vi "Close DSF Config Data.vi"(6 "version (no change)":T1, 8 "error in (no error)":errorcluster, 10 "write file if changed (T)":bool=TRUE, 11 "refnum":T2) -> (0 "error out":errorcluster, 3 "file path":path)   [LabVIEW 2017, in "DSF Configuration API.lvlib"]
doc: "Writes data to the platform-independent configuration file identified by <B>refnum</B> and then closes the reference to that file."
uses:
  DSF Configuration API.lvlib
  Controls/DSF Config Data RefNum.ctl
  Controls/Version Info.ctl
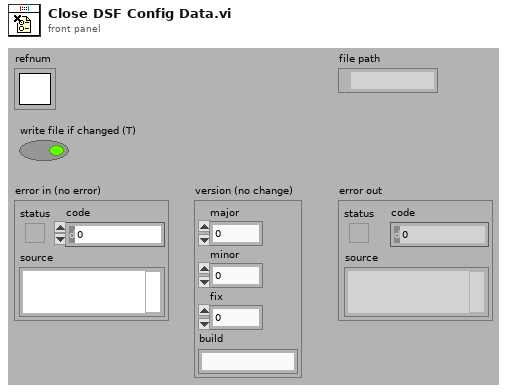
[diagram p1: front panel]
types:
  T1 = typedef "DSF Configuration API.lvlib/Version Info.ctl" = cluster{"major":u32, "minor":u32, "fix":u32, "build":string}
  T2 = typedef "DSF Configuration API.lvlib/DSF Config Data RefNum.ctl" = refnum<k1>
  T3 = typedef "DSF Configuration API.lvlib/Config Queue.ctl" = refnum<queue>
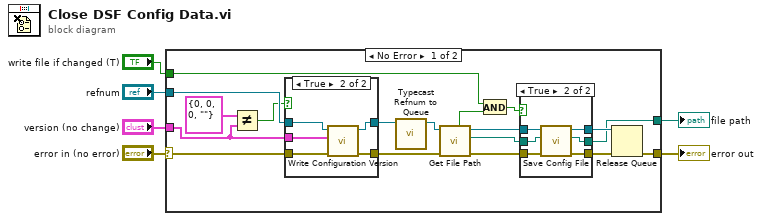
[diagram p0: block diagram]
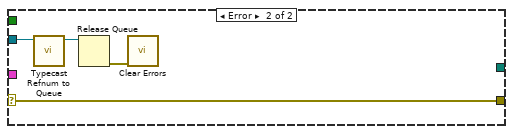
[diagram p4: hidden frame]
diagram:
  n1 = case shown="No Error" "error in (no error)" {
    selector: "error in (no error)" -> [w21 w44]
    tunnel: "refnum" -> [w11 w43]
    tunnel: "write file if changed (T)" -> [w23 _]
    tunnel: [w18 w44] -> w4
    tunnel: [w13 _] -> w3
    tunnel: "version (no change)" -> [w7 _]
    frame No Error {
      n2 = Not Equal?(x=T1 {"major"=0, "minor"=0, "fix"=0, "build"=""} ("version"), y=w7) -> (x != y?=w8:bool)
      n3 = case shown="True" w8 {
        tunnel: w21 -> [w25 w31]
        tunnel: [w25 w30] -> w12
        tunnel: w11 -> [w26 w29]
        tunnel: [w26 w28] -> w10
        tunnel: w7 -> [_ w27]
        frame False {
        }
        frame True {
          n4 = call "Write Configuration Version.vi"("error in (no error)"=w31, "Configuration Version"=w27, "refnum"=w29) -> ("error out"=w30:errorcluster, "refnum out"=w28:T2)  [unwired: 7 in]
        }
      }
      n5 = call "Typecast Refnum to Queue.vi"("refnum in"=w10) -> ("queue out"=w17:T3)  [unwired: 10 in]
      n6 = call "Get File Path.vi"("error in (no error)"=w12, "queue in"=w17) -> ("error out"=w15:errorcluster, "file path"=w14:path, "queue out"=w22:T3, "need update"=w16:bool)  [unwired: 1 in, 5 out]
      n7 = And(x=w23, y=w16) -> (x .and. y?=w24:bool)
      n8 = case shown="True" w24 {
        tunnel: w15 -> [w34 w40]
        tunnel: w22 -> [w33 w35]
        tunnel: [w34 w39] -> w19
        tunnel: [w33 w38] -> w20
        tunnel: w14 -> [w32 w37]
        tunnel: [w32 w36] -> w13
        frame False {
        }
        frame True {
          n9 = call "Save Config File.vi"("error in (no error)"=w40, "file path"=w37, "queue in"=w35) -> ("error out"=w39:errorcluster, "file path out"=w36:path, "queue out"=w38:T3)  [unwired: 6 out]
        }
      }
      n10 = Release Queue(queue=w20, error in (no error)=w19) -> (error out=w18:errorcluster)  [unwired: 1 in, 2 out]
    }
    frame Error {
      n11 = call "Typecast Refnum to Queue.vi"("refnum in"=w43) -> ("queue out"=w42:T3)  [unwired: 10 in]
      n12 = Release Queue(queue=w42) -> (error out=w41:errorcluster)  [unwired: 2 in, 2 out]
      n13 = call <vilib>:"Clear Errors.vi"("error in (no error)"=w41) -> ()  [unwired: 5 in, 2 out]
    }
  }
  "error out" <- w4
  "file path" <- w3
